vi "Example Graph - IAQIndex Callback.vi"(4 "IAQIndex":refnum<user-event>, 5 "Event Data":T1, 6 "Control Ref":refnum<k24>, 7 "Event Common Data":T2) -> ()   [LabVIEW 2010]
uses:
  C:/tf/play/labview/Tinkerforge.dll
  Tinkerforge.dll
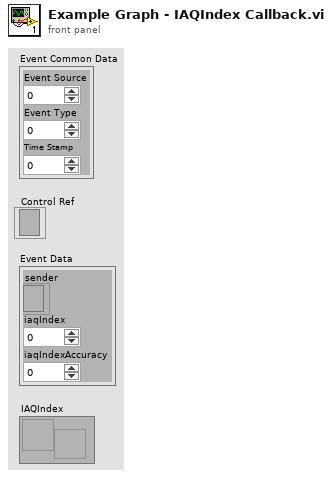
[diagram p1: front panel]
types:
  T1 = cluster{"sender":refnum<k24>, "iaqIndex":i32, "iaqIndexAccuracy":u8}
  T2 = cluster{"Event Source":i32, "Event Type":u32, "Time Stamp":u32}
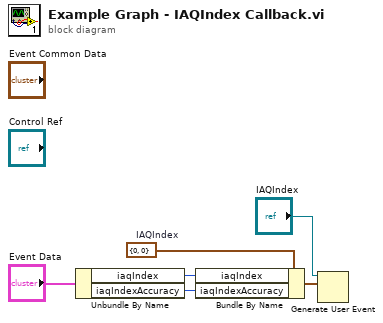
[diagram p0: block diagram]
diagram:
  w5 = cluster{"iaqIndex":i32, "iaqIndexAccuracy":u8} {"iaqIndex"=0, "iaqIndexAccuracy"=0}  # IAQIndex
  n1 = Unbundle By Name("Event Data") -> ("iaqIndex"=w4:i32, "iaqIndexAccuracy"=w3:u8)
  n2 = Bundle By Name(cluster=w5, "iaqIndex"=w4, "iaqIndexAccuracy"=w3) -> (w2:cluster{"iaqIndex":i32, "iaqIndexAccuracy":u8})
  n3 = Generate User Event(user event="IAQIndex", event data cluster=w2) -> ()  [unwired: 1 in, 2 out]
